vi "Write Meta Data.vi"(10 "Meta Data":string, 11 "Tree Data In":refnum<class "Tree Data.lvclass">) -> (3 "Tree Data Out":refnum<class "Tree Data.lvclass">)   [LabVIEW 2016, in "Tree Data.lvclass"]
doc: "Read the Meta Data associated with this Tree Data type."
uses:
  Tree Data.lvclass
  Tree Data.lvclass/Tree Data.ctl
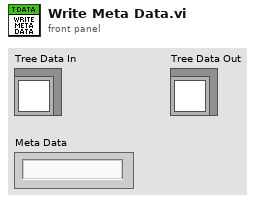
[diagram p1: front panel]
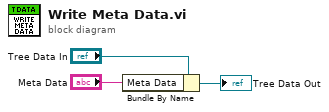
[diagram p0: block diagram]
diagram:
  n1 = Bundle By Name(cluster="Tree Data In", "Meta Data"="Meta Data") -> (→"Tree Data Out":refnum<class "Tree Data.lvclass">)
